vi "속도,조향각 PI제어(11.25).vi"() -> ()   [LabVIEW 2018]
panel:
  in  "Logging On/Off":bool
  in  "Logging 저장위치":path
  in  "전체 정지":bool
  out "최고조향각 인덱스":u16
  out "주행중 최대조향각[deg]":dbl
  out "최고속도 인덱스":u16
  out "Sub Control 사용":bool
  out "주행중 최대속도[m/s]":dbl
  out "알림자 활성화":bool
  out "Steer":dbl
  out "Speed":dbl
  out "Gear":dbl
  in  "조향각 출력 프로토콜":dbl
  in  "속도1 or 속도2":dbl
  in  "Sub Control 활성화":bool
  out "Main Control 이상감지":bool
  in  "Sub Control 정지":bool
  out "E-STOP":bool
  out "Manual Mode":bool
  out "시리얼 통신 속도":dbl
  out "시리얼 통신 이상감지":bool
  out "수렴 완료":bool
  out "5% 수렴시간":dbl
  out "목표 조향각 데이터가 들어오는가?":bool
  out "목표 속도 데이터가 들어오는가?":bool
  out "현재 조향각[deg]":dbl(knob) scale=-20.0..20.0
  out "목표 조향각[deg]":dbl(knob) scale=-20.0..20.0
  out "현재속도[m/s]":dbl(knob) scale=0.0..8.0
  out "목표속도[m/s]":dbl(knob) scale=0.0..8.0
  out "목표속도가 6 m/s가 넘는가?":bool
  out "목표속도가 음수인가?":bool
  out "error[%]":dbl
  out "강제변환 전 속도입력":dbl
  out "속도 제어기 이상":bool
  out "dt":dbl
  in  "Main Control 정지":bool
  # "주행 기록"
  # "제어성능 지표"
  # "첫 번째 작동에서만 측정된다."
  # "오류 점검(Main)"
  # "상태"
  # "Sub Control"
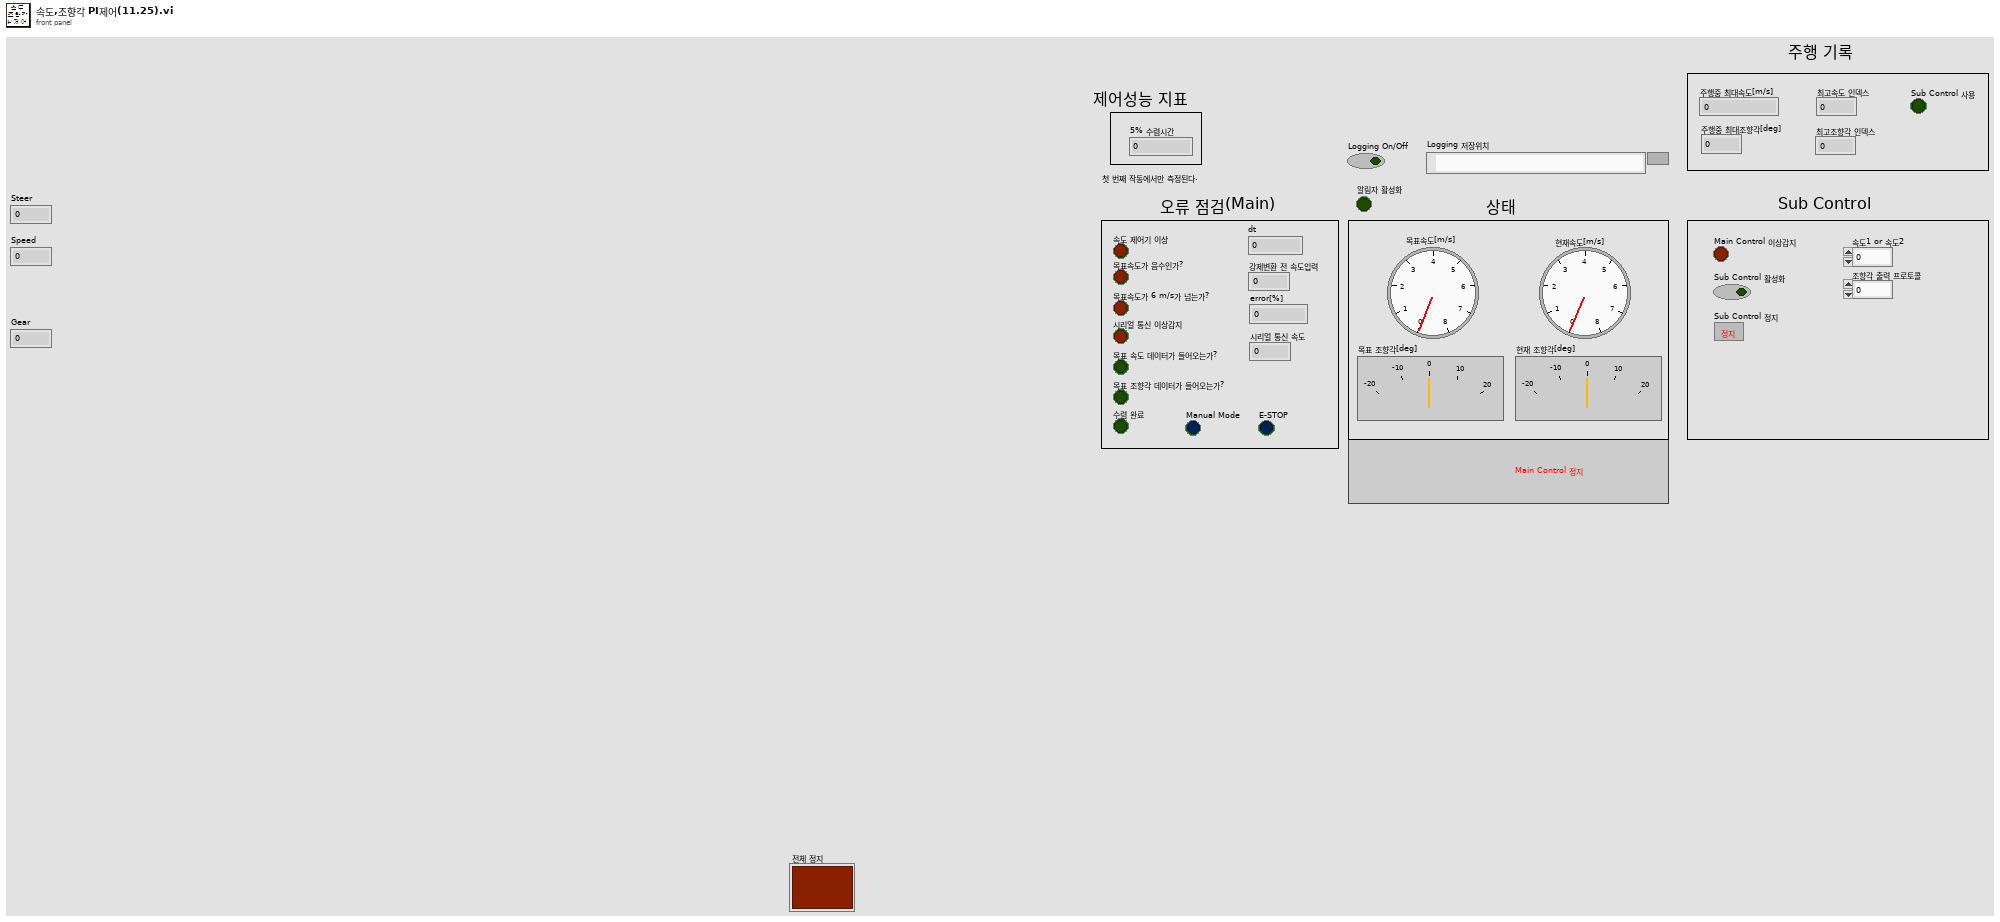
[diagram p1: front panel]
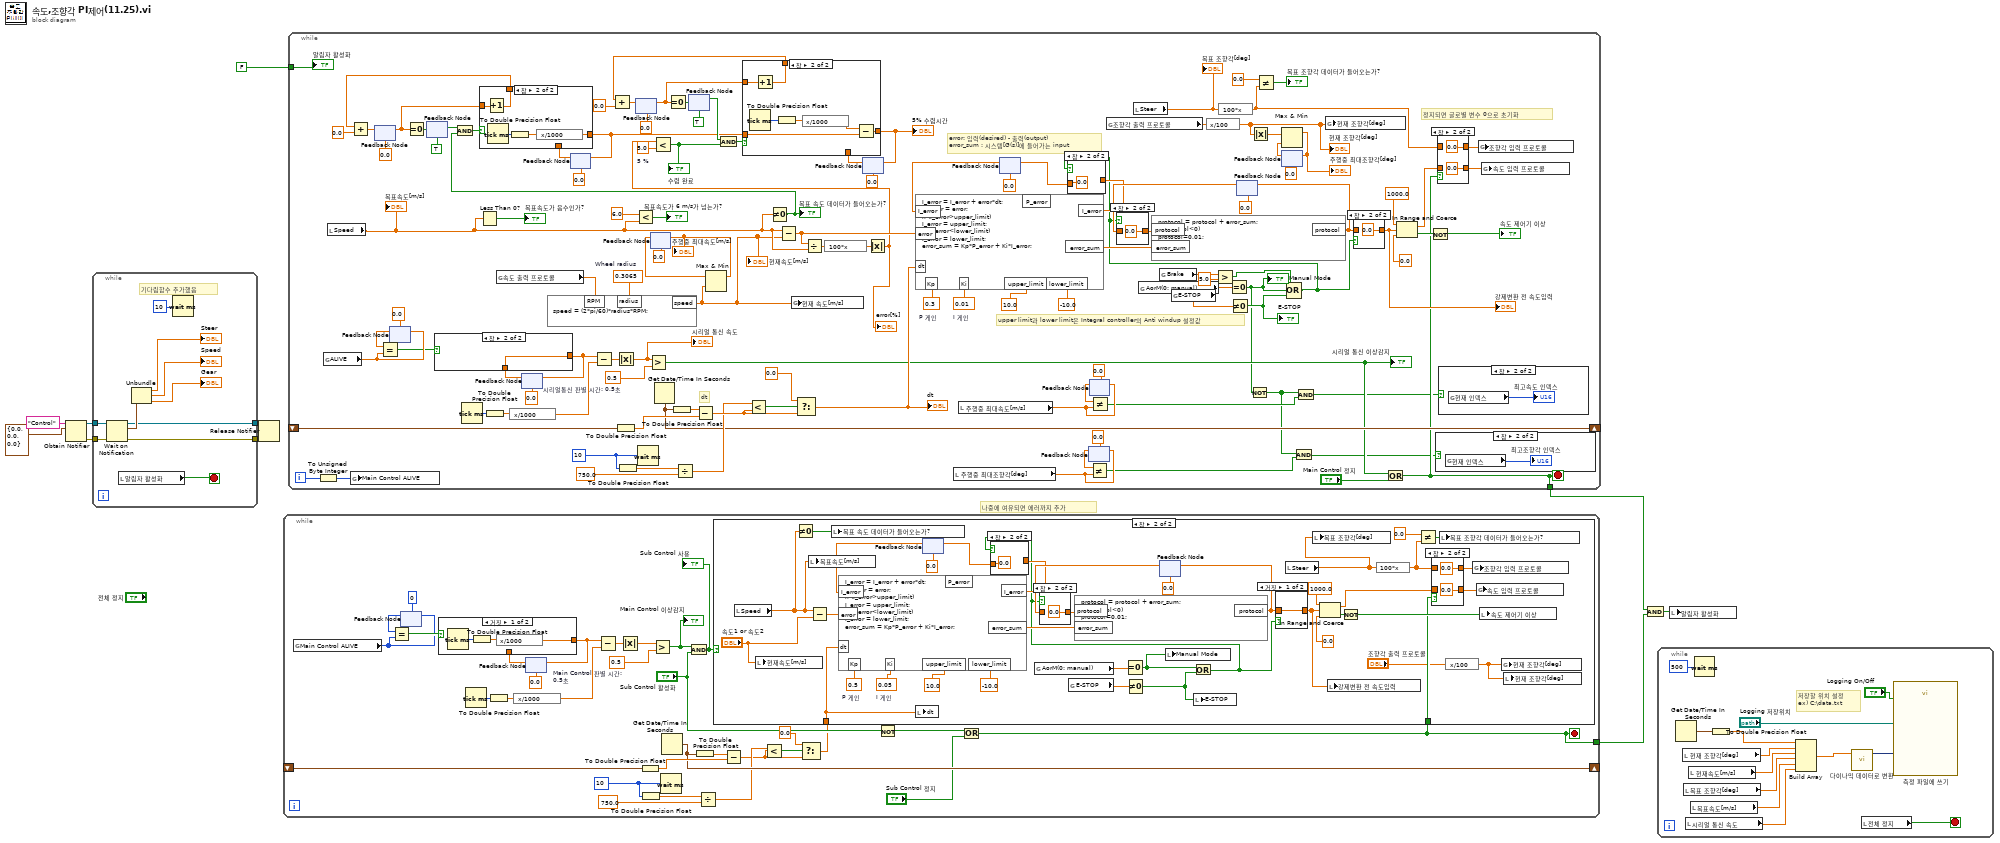
[diagram p0: block diagram]
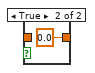
[diagram p7: hidden frame]
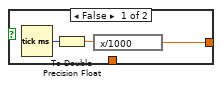
[diagram p13: hidden frame]
diagram:
  # "나중에 여유되면 에러까지 추가"
  n1 = Obtain Notifier(name (unnamed)="Control" ("이름(이름없음)"), notification data type=cluster{dbl, dbl, dbl} {0.0, 0.0, 0.0}) -> (notifier out=w8:refnum<notifier>, error out=w7:errorcluster)  [unwired: 2 in, 1 out]
  n2 = while {
    tunnel: w8 -> [w20]
    tunnel: w7 -> [w19]
    tunnel: [w14] -> w6
    tunnel: [w13] -> w5
    stop <- w11 stop-if-true
    # "기다림함수 추가했음"
    n3 = Wait on Notification(notifier=w20, error in (no error)=w19) -> (notifier out=w14:refnum<notifier>, notification=w18:cluster{dbl, dbl, dbl}, error out=w13:errorcluster)  [unwired: 2 in, 1 out]
    n4 = local read "알림자 활성화"() -> (w11:bool)
    n5 = Unbundle(w18) -> (→"Steer":dbl, →"Speed":dbl, →"Gear":dbl)
    n6 = Wait (ms)(milliseconds to wait=u32 10 ("대기 시간 (ms)")) -> ()  [unwired: 1 out]
  }
  n7 = Release Notifier(notifier=w6, error in (no error)=w5) -> ()  [unwired: 1 in, 3 out]
  n8 = while {
    shift-right: [w36] -> _
    shift-left: _ -> [w39]
    tunnel: [w21] -> w3
    stop <- w21 stop-if-true
    w33 = u32 10 ("대기 시간 (ms)")
    w43 = 0.5  # Main Control 판별 시간: 0.5초
    n9 = global read "글로벌 (11.23).vi" "Main Control ALIVE"() -> (w28:u8)
    n10 = feedback #1(u8 0 ("Dead Reckoning ALIVE")) -> (w51:u8)
    n11 = Equal?(x=w51, y=w28) -> (x = y?=w45:bool)
    n12 = feedback-in #1(w28) -> ()
    n13 = Tick Count (ms)() -> (millisecond timer value=w50:u32)
    n14 = To Double Precision Float(number=w50) -> (double precision float=w40:dbl)
    n15 = expression code="x/1000"(w40) -> (w42:dbl)
    n16 = feedback #2(0.0) -> (w49:dbl)
    n17 = case shown="거짓" w45 {
      tunnel: [w52 w55] -> w47
      tunnel: w49 -> [_ w55]
      frame False {
        n18 = Tick Count (ms)() -> (millisecond timer value=w53:u32)
        n19 = To Double Precision Float(number=w53) -> (double precision float=w54:dbl)
        n20 = expression code="x/1000"(w54) -> (w52:dbl)
      }
      frame True {
      }
    }
    n21 = feedback-in #2(w47) -> ()
    n22 = Subtract(x=w47, y=w42) -> (x-y=w46:dbl)
    n23 = Absolute Value(x=w46) -> (abs(x)=w44:dbl)
    n24 = To Double Precision Float(number=w39) -> (double precision float=w37:dbl)
    n25 = To Double Precision Float(number=w33) -> (double precision float=w35:dbl)
    n26 = Greater?(x=w44, y=w43) -> (0:w27:bool)
    "Main Control 이상감지" <- w27
    n27 = Wait (ms)(milliseconds to wait=w33) -> ()  [unwired: 1 out]
    n28 = Get Date/Time In Seconds() -> (seconds since 1Jan1904=w36:timestamp)
    n29 = And(x=w27, y="Sub Control 활성화") -> (x .and. y?=w26:bool)
    "Sub Control 사용" <- w26
    n30 = To Double Precision Float(number=w36) -> (double precision float=w38:dbl)
    n31 = Divide(x=w35, y=750.0) -> (x/y=w32:dbl)
    n32 = Subtract(x=w38, y=w37) -> (x-y=w29:dbl)
    n33 = Less?(x=w32, y=w29) -> (x < y?=w31:bool)
    n34 = Select(t=0.0, s=w31, f=w29) -> (s? t:f=w22:dbl)
    n35 = Not(x="Sub Control 활성화") -> (.not. x?=w24:bool)
    n36 = Or(x=w24, y="Sub Control 정지") -> (x .or. y?=w21:bool)
    n37 = case shown="참" w26 {
      tunnel: w22 -> [_ w59]
      tunnel: w21 -> [_ w66]
      frame False {
      }
      frame True {
        w90 = 0.05  # I 게인
        w91 = 0.5  # P 게인
        n38 = local read "Speed"() -> (w57:dbl)
        n39 = local write "현재속도[m/s]"("속도1 or 속도2") -> ()
        n40 = Not Equal To 0?(x=w57) -> (x != 0?=w58:bool)
        n41 = local write "목표속도[m/s]"(w57) -> ()
        n42 = Subtract(x=w57, y="속도1 or 속도2") -> (x-y=w76:dbl)
        n43 = local write "목표 속도 데이터가 들어오는가?"(w58) -> ()
        n44 = local write "dt"(w59) -> ()
        n45 = feedback #3(0.0 ("I_error")) -> (w93:dbl)
        n46 = formula code="I_error = I_error + error*dt;\nP_error = error;\nif (I_error>upper_limit)\nI_error = upper_limit;\nif (I_error<lower_limit)\nI_error = lower_limit;\nerror_sum = Kp*P_error + Ki*I_error;"("Kp"=w91, "Ki"=w90, "dt"=w59, "I_error"=w93, "error"=w76, "upper_limit"=10.0 ("입력 변수"), "lower_limit"=-10.0 ("입력 변수")) -> ("I_error"=w79:dbl, "error_sum"=w84:dbl)  [unwired: 1 out]
        n47 = global read "글로벌 (11.23).vi" "AorM(0: manual)"() -> (w83:dbl)
        n48 = global read "글로벌 (11.23).vi" "E-STOP"() -> (w77:dbl)
        n49 = Equal To 0?(x=w83) -> (x = 0?=w73:bool)
        n50 = Not Equal To 0?(x=w77) -> (x != 0?=w74:bool)
        n51 = feedback #4(0.0) -> (w80:dbl)
        n52 = local write "Manual Mode"(w73) -> ()
        n53 = Or(x=w73, y=w74) -> (x .or. y?=w75:bool)
        n54 = case shown="참" w75 {
          tunnel: w79 -> [w98 _]
          tunnel: [w98 0.0 ("I_error")] -> w78
          frame False {
          }
          frame True {
          }
        }
        n55 = feedback-in #3(w78) -> ()
        n56 = case shown="참" w75 {
          tunnel: w80 -> [w100 _]
          tunnel: [w100 0.0 ("목표 조향각[deg]")] -> w81
          frame False {
          }
          frame True {
          }
        }
        n57 = formula code="protocol = protocol + error_sum;\nif(protocol<0)\nprotocol=0.01;"("protocol"=w81, "error_sum"=w84) -> ("protocol"=w82:dbl)
        n58 = feedback-in #4(w82) -> ()
        n59 = local write "E-STOP"(w74) -> ()
        n60 = case shown="거짓" w75 {
          tunnel: w82 -> [w102 _]
          tunnel: [w102 0.0 ("목표 조향각[deg]")] -> w72
          frame False {
          }
          frame True {
          }
        }
        n61 = local read "Steer"() -> (w56:dbl)
        n62 = local write "목표 조향각[deg]"(w56) -> ()
        n63 = In Range and Coerce(upper limit=1000.0 ("상위 리미트"), x=w72, lower limit=0.0 ("하위 리미트")) -> (coerced(x)=w67:dbl, In Range?=w71:bool)
        n64 = local write "강제변환 전 속도입력"(w72) -> ()
        n65 = Not(x=w71) -> (.not. x?=w70:bool)
        n66 = expression code="100*x"(w56) -> (w63:dbl)
        n67 = Not Equal?(x=0.0, y=w63) -> (x != y?=w64:bool)
        n68 = case shown="참" w66 {
          tunnel: w63 -> [w95 _]
          tunnel: [w95 0.0 ("목표 조향각[deg]")] -> w69
          tunnel: [w94 0.0 ("상위 리미트")] -> w68
          tunnel: w67 -> [w94 _]
          frame False {
          }
          frame True {
          }
        }
        n69 = local write "목표 조향각 데이터가 들어오는가?"(w64) -> ()
        n70 = expression code="x/100"("조향각 출력 프로토콜") -> (w62:dbl)
        n71 = global write "글로벌 (11.23).vi" "조향각 입력 프로토콜"(w69) -> ()
        n72 = global write "글로벌 (11.23).vi" "속도 입력 프로토콜"(w68) -> ()
        n73 = local write "속도 제어기 이상"(w70) -> ()
        n74 = global write "글로벌 (11.23).vi" "현재 조향각[deg]"(w62) -> ()
        n75 = local write "현재 조향각[deg]"(w62) -> ()
      }
    }
  }
  n76 = while {
    shift-right: [w217] -> _
    shift-left: _ -> [w216]
    tunnel: FALSE -> [w132]
    tunnel: [w131] -> w2
    i -> [w136]
    stop <- w131 stop-if-true
    w147 = 0.5  # 시리얼통신 판별 시간: 0.5초
    w188 = 5.0  # 5 %
    w208 = 0.3065  # Wheel radius
    w211 = 0.01  # I 게인
    w212 = 0.3  # P 게인
    w218 = u32 10 ("대기 시간 (ms)")
    # "정지되면 글로별 변수 0으로 초기화"
    # "upper limit과 lower limit은 Integral controller의 Anti windup 설정값"
    # "error: 입력(desired) - 출력(output)\nerror_sum : 시스템[G(s)]에 들어가는 input"
    # "dt"
    n77 = To Unsigned Byte Integer(number=w136) -> (unsigned 8bit integer=w135:u8)
    n78 = global read "글로벌 (11.23).vi" "ALIVE"() -> (w158:dbl)
    n79 = local read "Speed"() -> (w134:dbl)
    "목표속도[m/s]" <- w134
    n80 = global write "글로벌 (11.23).vi" "Main Control ALIVE"(w135) -> ()
    n81 = feedback #5(0.0) -> (w176:dbl)
    n82 = feedback #6(0.0 ("ALIVE")) -> (w159:dbl)
    n83 = Equal?(x=w159, y=w158) -> (x = y?=w149:bool)
    n84 = feedback-in #6(w158) -> ()
    n85 = Equal To 0?(x=w176) -> (x = 0?=w180:bool)
    n86 = feedback-in #7(w180) -> ()
    n87 = feedback #7(TRUE) -> (w179:bool)
    n88 = Tick Count (ms)() -> (millisecond timer value=w155:u32)
    n89 = Less Than 0?(x=w134) -> (x < 0?=→"목표속도가 음수인가?":bool)
    n90 = To Double Precision Float(number=w155) -> (double precision float=w156:dbl)
    n91 = global read "글로벌 (11.23).vi" "속도 출력 프로토콜"() -> (w204:dbl)
    n92 = expression code="x/1000"(w156) -> (w151:dbl)
    n93 = feedback #8(0.0) -> (w154:dbl)
    n94 = case shown="참" w149 {
      tunnel: [w234 w237] -> w152
      tunnel: w154 -> [_ w237]
      frame False {
        n95 = Tick Count (ms)() -> (millisecond timer value=w235:u32)
        n96 = To Double Precision Float(number=w235) -> (double precision float=w236:dbl)
        n97 = expression code="x/1000"(w236) -> (w234:dbl)
      }
      frame True {
      }
    }
    n98 = feedback-in #8(w152) -> ()
    n99 = formula code="speed = (2*pi/60)*radius*RPM;"("radius"=w208, "RPM"=w204) -> ("speed"=w127:dbl)
    "현재속도[m/s]" <- w127
    n100 = feedback #9(0.0) -> (w164:dbl)
    n101 = Subtract(x=w152, y=w151) -> (x-y=w150:dbl)
    n102 = Absolute Value(x=w150) -> (abs(x)=w148:dbl)
    "시리얼 통신 속도" <- w148
    n103 = To Double Precision Float(number=w216) -> (double precision float=w225:dbl)
    n104 = To Double Precision Float(number=w218) -> (double precision float=w221:dbl)
    n105 = Less?(x=6.0, y=w134) -> (x < y?=→"목표속도가 6 m/s가 넘는가?":bool)
    n106 = feedback #10(0.0) -> (w168:dbl)
    n107 = Wait (ms)(milliseconds to wait=w218) -> ()  [unwired: 1 out]
    n108 = Greater?(x=w148, y=w147) -> (0:w145:bool)
    "시리얼 통신 이상감지" <- w145
    n109 = feedback #11(0.0 ("speed")) -> (w129:dbl)
    n110 = Get Date/Time In Seconds() -> (seconds since 1Jan1904=w217:timestamp)
    n111 = Equal To 0?(x=w168) -> (x = 0?=w172:bool)
    n112 = To Double Precision Float(number=w217) -> (double precision float=w224:dbl)
    n113 = Divide(x=w221, y=750.0) -> (x/y=w219:dbl)
    n114 = feedback #12(TRUE) -> (w166:bool)
    n115 = feedback-in #12(w172) -> ()
    n116 = Subtract(x=w224, y=w225) -> (x-y=w222:dbl)
    n117 = Max & Min(x=w129, y=w127) -> (max(x,y)=w128:dbl)  [unwired: 1 out]
    "주행중 최대속도[m/s]" <- w128
    n118 = feedback-in #11(w128) -> ()
    n119 = Less?(x=w219, y=w222) -> (x < y?=w223:bool)
    n120 = Not Equal To 0?(x=w134) -> (x != 0?=w183:bool)
    "목표 속도 데이터가 들어오는가?" <- w183
    n121 = And(x=w179, y=w183) -> (x .and. y?=w185:bool)
    n122 = case shown="참" w185 {
      tunnel: [w238 w242] -> w165
      tunnel: [w239 w241] -> w181
      tunnel: w176 -> [w239 w240]
      tunnel: w164 -> [w238 _]
      frame False {
      }
      frame True {
        n123 = Increment(x=w240) -> (x+1=w241:dbl)
        n124 = Tick Count (ms)() -> (millisecond timer value=w244:u32)
        n125 = To Double Precision Float(number=w244) -> (double precision float=w243:dbl)
        n126 = expression code="x/1000"(w243) -> (w242:dbl)
      }
    }
    n127 = Add(x=w181, y=0.0) -> (x+y=w177:dbl)
    n128 = feedback-in #5(w177) -> ()
    n129 = feedback-in #9(w165) -> ()
    n130 = Subtract(x=w134, y=w127) -> (x-y=w190:dbl)
    n131 = global write "글로벌 (11.23).vi" "현재 속도[m/s]"(w127) -> ()
    n132 = Select(t=0.0, s=w223, f=w222) -> (s? t:f=w207:dbl)
    "dt" <- w207
    n133 = Divide(x=w190, y=w134) -> (x/y=w189:dbl)
    n134 = expression code="100*x"(w189) -> (w187:dbl)
    n135 = feedback #13(0.0) -> (w161:dbl)
    n136 = Absolute Value(x=w187) -> (abs(x)=w186:dbl)
    "error[%]" <- w186
    n137 = Less?(x=w186, y=w188) -> (x < y?=w174:bool)
    "수렴 완료" <- w174
    n138 = And(x=w166, y=w174) -> (x .and. y?=w184:bool)
    n139 = case shown="참" w184 {
      tunnel: w165 -> [_ w253]
      tunnel: [w245 w252] -> w162
      tunnel: w168 -> [w246 w248]
      tunnel: [w246 w247] -> w167
      tunnel: w161 -> [w245 _]
      frame False {
      }
      frame True {
        n140 = Tick Count (ms)() -> (millisecond timer value=w251:u32)
        n141 = Increment(x=w248) -> (x+1=w247:dbl)
        n142 = To Double Precision Float(number=w251) -> (double precision float=w250:dbl)
        n143 = expression code="x/1000"(w250) -> (w249:dbl)
        n144 = Subtract(x=w249, y=w253) -> (x-y=w252:dbl)
      }
    }
    "5% 수렴시간" <- w162
    n145 = Add(x=w167, y=0.0) -> (x+y=w170:dbl)
    n146 = feedback-in #10(w170) -> ()
    n147 = feedback-in #13(w162) -> ()
    n148 = local read "주행중 최대조향각[deg]"() -> (w113:dbl)
    n149 = local read "주행중 최대속도[m/s]"() -> (w126:dbl)
    n150 = feedback #14(0.0 ("I_error")) -> (w214:dbl)
    n151 = formula code="I_error = I_error + error*dt;\nP_error = error;\nif (I_error>upper_limit)\nI_error = upper_limit;\nif (I_error<lower_limit)\nI_error = lower_limit;\nerror_sum = Kp*P_error + Ki*I_error;"("Kp"=w212, "Ki"=w211, "dt"=w207, "I_error"=w214, "error"=w190, "upper_limit"=10.0 ("입력 변수"), "lower_limit"=-10.0 ("입력 변수")) -> ("I_error"=w139:dbl, "error_sum"=w196:dbl)  [unwired: 1 out]
    n152 = feedback #15(0.0 ("주행중 최대속도[m/s]")) -> (w114:dbl)
    n153 = feedback-in #15(w113) -> ()
    n154 = feedback-in #16(w126) -> ()
    n155 = feedback #16(0.0 ("주행중 최대속도[m/s]")) -> (w125:dbl)
    n156 = Not Equal?(x=w114, y=w113) -> (x != y?=w112:bool)
    n157 = Not Equal?(x=w125, y=w126) -> (x != y?=w121:bool)
    n158 = global read "글로벌 (11.23).vi" "조향각 출력 프로토콜"() -> (w203:dbl)
    n159 = local read "Steer"() -> (w133:dbl)
    "목표 조향각[deg]" <- w133
    n160 = global read "글로벌 (11.23).vi" "AorM(0: manual)"() -> (w144:dbl)
    n161 = global read "글로벌 (11.23).vi" "Brake"() -> (w106:dbl)
    n162 = global read "글로벌 (11.23).vi" "E-STOP"() -> (w137:dbl)
    n163 = expression code="x/100"(w203) -> (w117:dbl)
    "현재 조향각[deg]" <- w117
    n164 = Greater?(x=w106, y=5.0) -> (0:w104:bool)
    n165 = expression code="100*x"(w133) -> (w195:dbl)
    n166 = Equal To 0?(x=w144) -> (x = 0?=w108:bool)
    "Manual Mode" <- w108
    n167 = Not Equal To 0?(x=w137) -> (x != 0?=w109:bool)
    "E-STOP" <- w109
    n168 = feedback #17(0.0) -> (w140:dbl)
    n169 = Not(x=w108) -> (.not. x?=w111:bool)
    n170 = Absolute Value(x=w117) -> (abs(x)=w116:dbl)
    n171 = Not Equal?(x=0.0, y=w195) -> (x != y?=→"목표 조향각 데이터가 들어오는가?":bool)
    n172 = feedback #18(0.0) -> (w120:dbl)
    n173 = Max & Min(x=w116, y=w120) -> (max(x,y)=w119:dbl)  [unwired: 1 out]
    "주행중 최대조향각[deg]" <- w119
    n174 = feedback-in #18(w119) -> ()
    n175 = Compound Arithmetic op=OR ("복합 연산")(w104, w108, w109) -> (w107:bool)
    n176 = case shown="참" w107 {
      tunnel: w139 -> [w228 _]
      tunnel: [w228 0.0 ("I_error")] -> w138
      frame False {
      }
      frame True {
      }
    }
    n177 = feedback-in #14(w138) -> ()
    n178 = case shown="참" w107 {
      tunnel: w140 -> [w230 _]
      tunnel: [w230 0.0 ("목표 조향각[deg]")] -> w141
      frame False {
      }
      frame True {
      }
    }
    n179 = formula code="protocol = protocol + error_sum;\nif(protocol<0)\nprotocol=0.01;"("protocol"=w141, "error_sum"=w196) -> ("protocol"=w142:dbl)
    n180 = feedback-in #17(w142) -> ()
    n181 = And(x=w111, y=w112) -> (x .and. y?=w110:bool)
    n182 = And(x=w111, y=w121) -> (x .and. y?=w122:bool)
    n183 = global write "글로벌 (11.23).vi" "현재 조향각[deg]"(w117) -> ()
    n184 = case shown="참" w107 {
      tunnel: w142 -> [w232 _]
      tunnel: [w232 0.0 ("목표 조향각[deg]")] -> w143
      frame False {
      }
      frame True {
      }
    }
    "강제변환 전 속도입력" <- w143
    n185 = Or(x=w145, y="Main Control 정지") -> (x .or. y?=w131:bool)
    n186 = In Range and Coerce(upper limit=1000.0 ("상위 리미트"), x=w143, lower limit=0.0 ("하위 리미트")) -> (coerced(x)=w192:dbl, In Range?=w191:bool)
    n187 = Not(x=w191) -> (.not. x?=→"속도 제어기 이상":bool)
    n188 = case shown="참" w110 {
      frame False {
      }
      frame True {
        n189 = global read "글로벌 (11.23).vi" "현재 인덱스"() -> (→"최고조향각 인덱스":u16)
      }
    }
    n190 = case shown="참" w131 {
      tunnel: w195 -> [w255 _]
      tunnel: [w255 0.0 ("목표 조향각[deg]")] -> w194
      tunnel: [w254 0.0 ("상위 리미트")] -> w193
      tunnel: w192 -> [w254 _]
      frame False {
      }
      frame True {
      }
    }
    n191 = case shown="참" w122 {
      frame False {
      }
      frame True {
        n192 = global read "글로벌 (11.23).vi" "현재 인덱스"() -> (→"최고속도 인덱스":u16)
      }
    }
    n193 = global write "글로벌 (11.23).vi" "조향각 입력 프로토콜"(w194) -> ()
    n194 = global write "글로벌 (11.23).vi" "속도 입력 프로토콜"(w193) -> ()
    "알림자 활성화" <- w132
  }
  n195 = And(x=w2, y=w3) -> (x .and. y?=w1:bool)
  n196 = while {
    stop <- w263 stop-if-true
    # "저장할 위치 설정\nex) C:\\data.txt"
    n197 = Get Date/Time In Seconds() -> (seconds since 1Jan1904=w265:timestamp)
    n198 = local read "현재 조향각[deg]"() -> (w262:dbl)
    n199 = local read "목표 조향각[deg]"() -> (w260:dbl)
    n200 = local read "시리얼 통신 속도"() -> (w258:dbl)
    n201 = local read "현재속도[m/s]"() -> (w261:dbl)
    n202 = local read "목표속도[m/s]"() -> (w259:dbl)
    n203 = Wait (ms)(milliseconds to wait=u32 500 ("대기 시간 (ms)")) -> ()  [unwired: 1 out]
    n204 = To Double Precision Float(number=w265) -> (double precision float=w264:dbl)
    n205 = Build Array(w264, w262, w261, w260, w259, w258) -> (w266:dbl[])
    n206 = call "다이나믹 데이터로 변환"("Array"=w266) -> ("Dynamic Data Type"=w269:dynamicdata)  [unwired: 3 in]
    n207 = local read "전체 정지"() -> (w263:bool)
    n208 = call "측정 파일에 쓰기"("Signals"=w269, "Enable"="Logging On/Off", "Filename"="Logging 저장위치") -> ()  [unwired: 14 in, 3 out]
  }
  n209 = local write "알림자 활성화"(w1) -> ()
